vi "V,A_to_temp,res.vi"(10 "Current":dbl[](array[numeric]), 11 "Volt":dbl[](array[numeric])) -> (2 "Temp":dbl[](array[numeric]), 3 "Res":dbl[](array[numeric]))   [LabVIEW 2022 SP3]
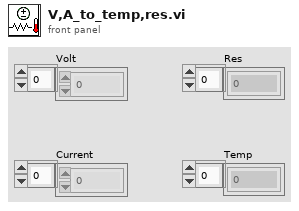
[diagram p1: front panel]
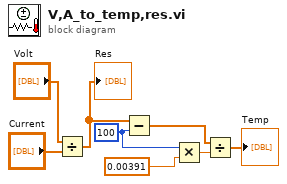
[diagram p0: block diagram]
diagram:
  w2 = 100 ("mean")
  n1 = Divide(x="Volt", y="Current") -> (x/y=w8:dbl[])
  "Res" <- w8
  n2 = Subtract(x=w8, y=w2) -> (x-y=w1:dbl[])
  n3 = Multiply(x=w2, y=0.00391) -> (x*y=w5:dbl)
  n4 = Divide(x=w1, y=w5) -> (x/y=→"Temp":dbl[])
